vi "get object by name.vi"(8 "error in (no error)":errorcluster, 10 "Name":path, 11 "system object in":refnum<class "system object.lvclass">) -> (0 "error out":errorcluster, 1 "Found":bool, 2 "Target object":refnum<class "system object.lvclass">, 3 "system object out":refnum<class "system object.lvclass">)   [LabVIEW 2020, in "system object.lvclass"]
uses:
  system object.lvclass
  system object.lvclass/system object.ctl
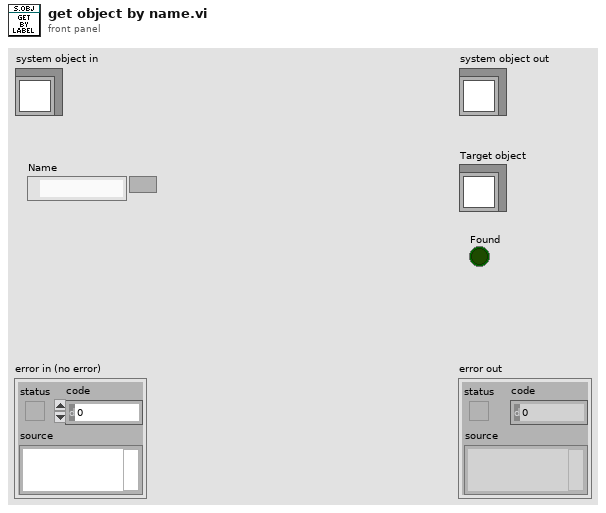
[diagram p1: front panel]
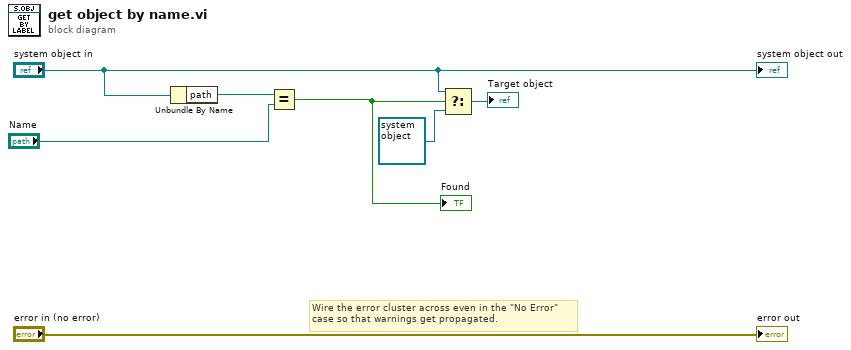
[diagram p0: block diagram]
diagram:
  # "Wire the error cluster across even in the \"No Error\"\ncase so that warnings get propagated."
  n1 = Unbundle By Name("system object in") -> ("path"=w6:path)
  n2 = Equal?(x=w6, y="Name") -> (x = y?=w4:bool)
  "Found" <- w4
  n3 = Select(t="system object in", s=w4, f=refnum<class "system object.lvclass"> refnum) -> (s? t:f=→"Target object":refnum<class "system object.lvclass">)
  "error out" <- "error in (no error)"
  "system object out" <- "system object in"
